vi "Mask Image.vi"(1 "Image Name Out":string="untitled", 4 "Image Name":string="untitled", 5 "Color Plane":i32(ring)=1 items=["Red", "Green", "Blue", "Hue", "Saturation", "Luminance", "Value", "Intensity"], 6 "Background Value (0)":i32, 7 "Rectangle":T2 {"Rotation" min=-90.0 max=90.0 step=1.0 format="%.2f"; "Left" scale=0.0..1024.0; "Right" scale=0.0..1024.0}, 8 "error in (no error)":errorcluster, 9 "Filling Value (255)":i32=255, 10 "Image Src":T1, 11 "Image Model":T1) -> (0 "error out":errorcluster, 2 "Coordinates out of space?":bool, 3 "Masked_Image":T1)   [LabVIEW 2017]
uses:
  <vilib>/vision/Image Controls.llb/IMAQ Image.ctl
  <vilib>/vision/NI_Vision_Development_Module.lvlib
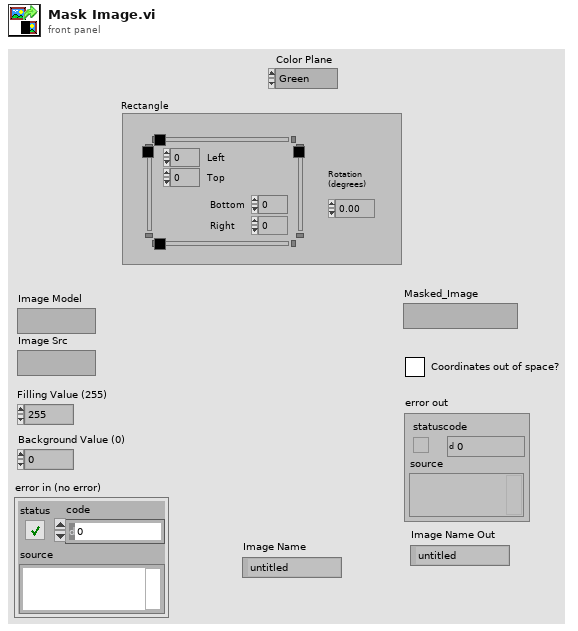
[diagram p1: front panel]
types:
  T1 = typedef "IMAQ Image.ctl" = refnum<image>
  T2 = typedef "IMAQ Rectangle" = cluster{"Left":i32, "Top":i32, "Right":i32, "Bottom":i32, "Rotation":dbl}
  T3 = typedef "Image Type" = u32
  T4 = typedef "ROI Descriptor" = cluster{"Global Rectangle":i32[], "Contours":cluster{"ID":enum32{"External", "Internal"}, "Type":u32, "Coordinates":i32[]}[]}
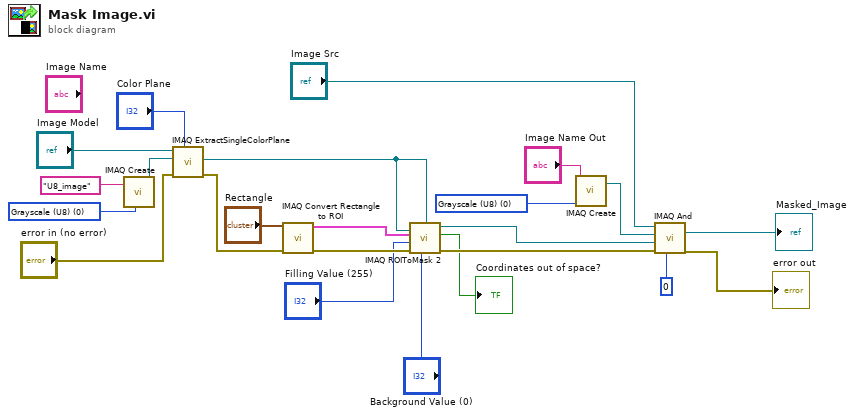
[diagram p0: block diagram]
diagram:
  w13 = T3 0 items=["Grayscale (U8)", "Grayscale (I16)", "Grayscale (SGL)", "Complex (CSG)", "RGB (U32)", "HSL (U32)", "RGB (U64)", "Grayscale (U16)"] ("Image Type")
  w19 = T3 0 items=["Grayscale (U8)", "Grayscale (I16)", "Grayscale (SGL)", "Complex (CSG)", "RGB (U32)", "HSL (U32)", "RGB (U64)", "Grayscale (U16)"] ("Image Type")
  n1 = call "IMAQ Create"("Image Name"="U8_image", "Image Type"=w13) -> ("New Image"=w12:T1)  [unwired: 3 in, 1 out]
  n2 = call "IMAQ ExtractSingleColorPlane"("Color Plane"="Color Plane", "error in (no error)"="error in (no error)", "Image Dst"=w12, "Image Src"="Image Model") -> ("error out"=w3:errorcluster, "Image Dst Out"=w15:T1)  [unwired: 6 in]
  n3 = call "IMAQ Convert Rectangle to ROI"("error in (no error)"=w3, "Rectangle"="Rectangle") -> ("error out"=w23:errorcluster, "ROI Descriptor"=w17:T4)  [unwired: 7 in]
  n4 = call "IMAQ ROIToMask 2"("Background Value (0)"="Background Value (0)", "Image Model"=w15, "error in (no error)"=w23, "Filling Value (255)"="Filling Value (255)", "ROI Descriptor"=w17, "Image"=w15) -> ("error out"=w21:errorcluster, "Coordinates out of space?"=→"Coordinates out of space?":bool, "Image Out"=w16:T1)  [unwired: 3 in]
  n5 = call "IMAQ Create"("Image Name"="Image Name Out", "Image Type"=w19) -> ("New Image"=w18:T1)  [unwired: 3 in, 1 out]
  n6 = call "IMAQ And"("Constant"=i64 0, "error in (no error)"=w21, "Image Src B"=w16, "Image Dst"=w18, "Image Src A"="Image Src") -> ("error out"=→"error out":errorcluster, "Image Dst Out"=→"Masked_Image":T1)  [unwired: 5 in]
